vi "ExSubCollectDisplayStoreCoolSnaptest.vi"(0 "Handle Cluster":T1, 1 "session ID":u64, 2 "Display Title":string, 3 "Store flag":i8, 5 "error in (no error)":errorcluster) -> (6 "Handle Cluster Out":T1, 7 "got frame":u32, 8 "error out":errorcluster)   [LabVIEW 2015]
uses:
  <vilib>/Enthought/Python Integration Toolkit/Python Integration Toolkit.lvlib
panel:
  out "z position 2":dbl
  out "z position":dbl
  # "ExSubCollectDisplayStoreCoolSnap:\nThis sub-VI checks to see if data has arrived from camera,\nif so it then puts it in image object and displays it. If store \nswitch is set it will also store it."
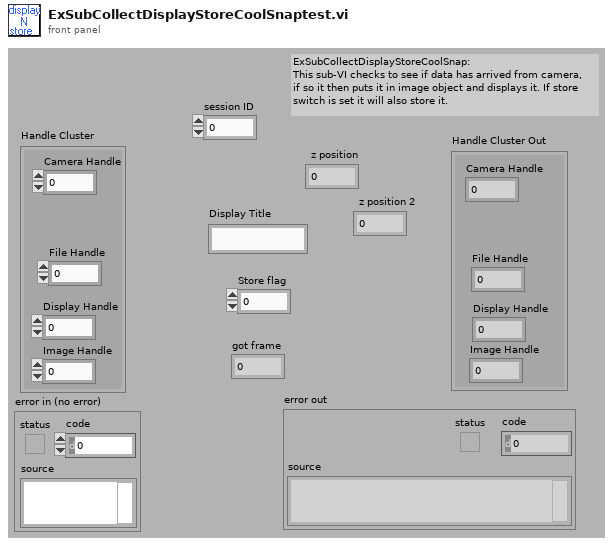
[diagram p1: front panel]
types:
  T1 = cluster{"Camera Handle":u32, "File Handle":u32, "Display Handle":u32, "Image Handle":u32}
  T2 = typedef "Python Integration Toolkit.lvlib/Python Objects.ctl" = variant
  T3 = typedef "Python Integration Toolkit.lvlib/Session ID.ctl" = u64
  T4 = cluster{"Camera Handle":u32, "File Handle":u32, "Display Handle":u32, "Data Handle":u32}
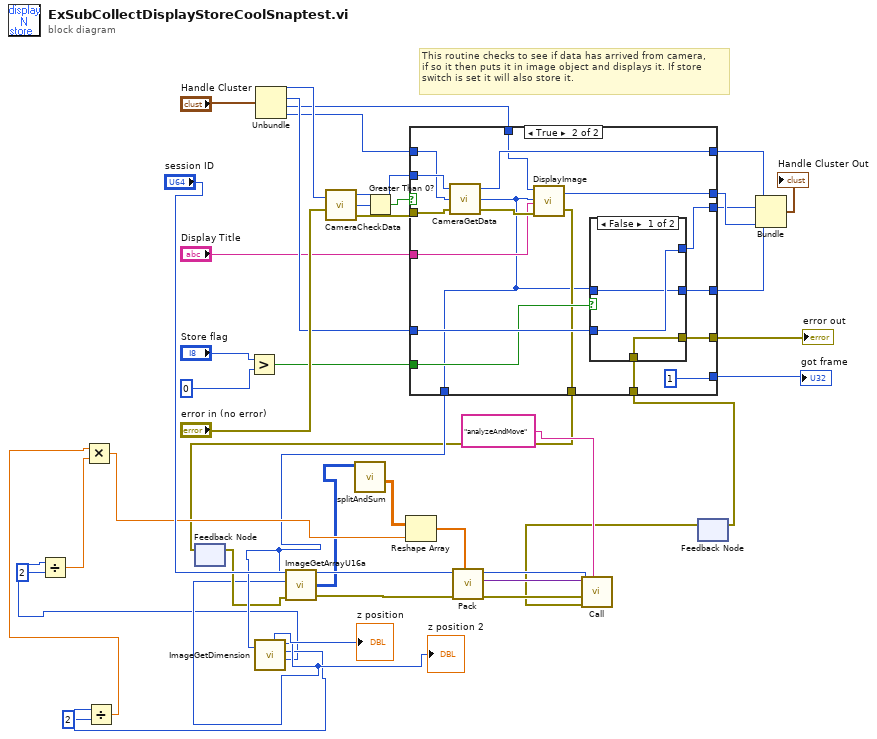
[diagram p0: block diagram]
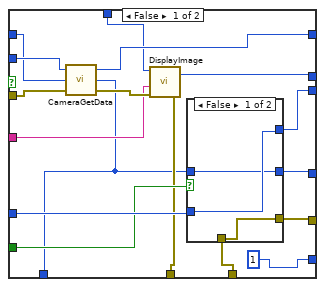
[diagram p2: hidden frame]
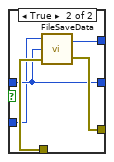
[diagram p3: hidden frame]
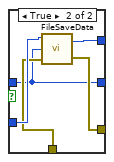
[diagram p4: hidden frame]
diagram:
  # "This routine checks to see if data has arrived from camera,\nif so it then puts it in image object and displays it. If store \nswitch is set it will also store it."
  n1 = feedback #1() -> (w14:errorcluster)  [unwired: 1 in]
  n2 = Greater?(x="Store flag", y=0) -> (0:w32:bool)
  n3 = Unbundle("Handle Cluster") -> ("Camera Handle"=w37:u32, "File Handle"=w31:u32, "Display Handle"=w30:u32, "Image Handle"=w29:u32)
  n4 = call <userlib>:"CameraCheckData.vi"("Camera Handle"=w37, "error in"="error in (no error)") -> ("Camera Handle"=w42:u32, "Number Of Frames Available"=w19:i32, "error out"=w41:errorcluster)
  n5 = Greater Than 0?(x=w19) -> (x > 0?=w18:bool)
  n6 = feedback #2() -> (w10:errorcluster)  [unwired: 1 in]
  n7 = case shown="True" w18 {
    tunnel: w42 -> [w60 w86]
    tunnel: w41 -> [w58 w85]
    tunnel: w29 -> [w59 w82]
    tunnel: w30 -> [w56 w81]
    tunnel: [w57 w84] -> w38
    tunnel: "Display Title" -> [w55 w80]
    tunnel: w31 -> [w54 w79]
    tunnel: [w46 w78] -> w36
    tunnel: [w49 w77] -> w39
    tunnel: [w47 w76] -> w35
    tunnel: w32 -> [w53 w75]
    tunnel: [w51 w74] -> w15
    tunnel: w10 -> [w50 w73]
    tunnel: [w45 w70] -> w16
    tunnel: [1 1] -> w24
    tunnel: [w48 w72] -> w23
    frame False {
      (unwired) 0
      n8 = call <userlib>:"CameraGetData.vi"("error in"=w58, "Data Handle"=w59, "Camera Handle"=w60) -> ("error out"=w61:errorcluster, "Data Handle"=w45:u32, "Camera Handle"=w57:u32)
      n9 = call <userlib>:"DisplayImage.vi"("error in"=w61, "Title"=w55, "Display Handle"=w56) -> ("error out"=w51:errorcluster, "Display Handle"=w46:u32)  [unwired: 1 in]
      n10 = case shown="False" w53 {
        tunnel: [w64 w65] -> w48
        tunnel: w50 -> [w63 w69]
        tunnel: w54 -> [w64 w66]
        tunnel: [w63 w68] -> w49
        tunnel: w45 -> [w62 w67]
        tunnel: [w62 w67] -> w47
        frame False {
        }
        frame True {
          n11 = call <userlib>:"FileSaveData.vi"("error in"=w69, "Image Handle"=w67, "File Handle"=w66) -> ("error out"=w68:errorcluster, "File Handle"=w65:u32)
        }
      }
    }
    frame True {
      n12 = call <userlib>:"CameraGetData.vi"("error in"=w85, "Data Handle"=w82, "Camera Handle"=w86) -> ("error out"=w83:errorcluster, "Data Handle"=w70:u32, "Camera Handle"=w84:u32)
      n13 = call <userlib>:"DisplayImage.vi"("error in"=w83, "Title"=w80, "Image Handle"=w70, "Display Handle"=w81) -> ("error out"=w74:errorcluster, "Display Handle"=w78:u32)
      n14 = case shown="False" w75 {
        tunnel: [w89 w94] -> w72
        tunnel: w79 -> [w89 w92]
        tunnel: [w88 w93] -> w77
        tunnel: [w87 w90] -> w76
        tunnel: w73 -> [w88 w91]
        tunnel: w70 -> [w87 w90]
        frame False {
        }
        frame True {
          n15 = call <userlib>:"FileSaveData.vi"("error in"=w91, "Image Handle"=w90, "File Handle"=w92) -> ("error out"=w93:errorcluster, "File Handle"=w94:u32)
        }
      }
    }
  }
  "error out" <- w39
  "got frame" <- w24
  n16 = feedback-in #1(w15) -> ()
  n17 = call <userlib>:"ImageGetDimension.vi"("Image Handle"=w16) -> ("Z dimension"=→"z position":u32, "Image Handle"=w13:u32, "X dimension"=w4:u32, "Y dimension"=w3:u32)  [unwired: 1 in, 2 out]
  "z position 2" <- w13
  n18 = Divide(x=w3, y=u32 2) -> (x/y=w5:dbl)
  n19 = Divide(x=w4, y=u32 2) -> (x/y=w6:dbl)
  n20 = Multiply(x=w6, y=w5) -> (x*y=w20:dbl)
  n21 = call <userlib>:"ImageGetArrayU16a.vi"("error in"=w14, "Z position"=w13, "Data Handle"=w16) -> ("error out"=w12:errorcluster, "Array uint 16"=w9:u16[][])  [unwired: 1 in, 1 out]
  n22 = call "splitAndSum.vi"("Real Matrix"=w9) -> ("Array"=w7:dbl[][])  [unwired: 8 in, 2 out]
  n23 = Reshape Array(w7, w20) -> (w8:dbl[])
  n24 = call <vilib>:"Pack.vi"("Argument"=w8, "error in (no error)"=w12, "Session ID"="session ID") -> ("error out"=w28:errorcluster, "Python Object References Out"=w27:T2, "Session ID out"=w26:T3)  [unwired: 6 in]
  n25 = call <vilib>:"Call.vi"("Function or Method Name"="analyzeAndMove", "error in (no error)"=w28, "Python Object References In"=w27, "Session ID"=w26) -> ("error out"=w11:errorcluster)  [unwired: 5 in, 2 out]
  n26 = feedback-in #2(w11) -> ()
  n27 = Bundle("Camera Handle"=w38, "File Handle"=w23, "Display Handle"=w36, "Data Handle"=w35) -> (→"Handle Cluster Out":T4)  [unwired: 1 in]
